vi "ixon get one frame - SubVI.vi"(4 "error in":errorcluster, 5 "Image Height":i32, 6 "Image Width":i32, 7 "Image In":T1) -> (0 "error out":errorcluster, 1 "Image Out":T1)   [LabVIEW 2014]
doc: "Waits till ready and then retireves on frame from an andor camera that has been previously started running a continuous acquisiiton. Uses the GetNewData16 library function."
uses:
  ATMCD32D.DLL
  <vilib>/vision/Image Controls.llb/IMAQ Image.ctl
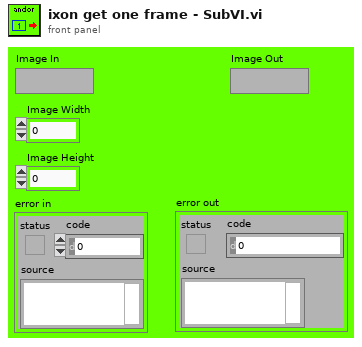
[diagram p1: front panel]
types:
  T1 = typedef "IMAQ Image.ctl" = refnum<image>
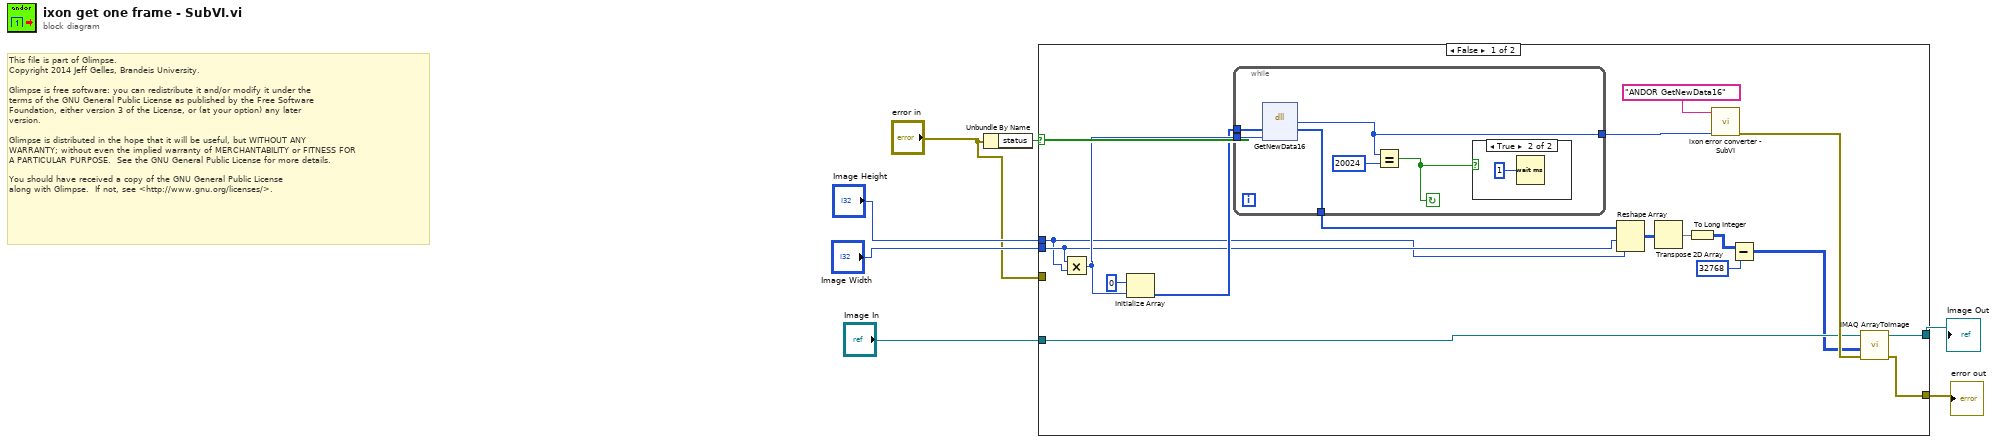
[diagram p0: block diagram]
diagram:
  # "This file is part of Glimpse. \nCopyright 2014 Jeff Gelles, Brandeis University.    \n\nGlimpse is free software: you can redistribute it and/or modify it under the \nterms of the GNU General Public License as published by the Free Software \nFoundation, either version 3 of the License, or (at your option) any later \nversion.\n\nGlimpse is distributed in the hope that it will be useful, but WITHOUT ANY \nWARRANTY; without even the implied warranty of MERCHANTABILITY or FITNESS FOR \nA PARTICULAR PURPOSE.  See the GNU General Public License for more details.\n\nYou should have received a copy of the GNU General Public License\nalong with Glimpse.  If not, see <http://www.gnu.org/licenses/>."
  n1 = Unbundle By Name("error in") -> ("status"=w3:bool)
  n2 = case shown="False" w3 {
    tunnel: "Image Height" -> [w8 _]
    tunnel: "Image Width" -> [w9 _]
    tunnel: "error in" -> [_ w33]
    tunnel: [w17 w33] -> w5
    tunnel: [w15 w32] -> w2
    tunnel: "Image In" -> [w14 w32]
    frame False {
      n3 = Multiply(x=w9, y=w8) -> (x*y=w19:i32)
      n4 = Initialize Array "Initialize Array"(u16 0, w19) -> (w13:u16[])
      n5 = while {
        tunnel: w13 -> [w30]
        tunnel: w19 -> [w29]
        tunnel: [w28] -> w23
        tunnel: [w27] -> w22
        stop <- w25 continue-if-true
        n6 = dll-call lib="ATMCD32D.DLL" fn="GetNewData16" label="Call Library Function\nGetNew data 16"(w30, w29) -> ("return type"=w27:u32, w28:u16[])  [unwired: 4 in, 2 out]
        n7 = Equal?(x=w27, y=u32 20024) -> (x = y?=w25:bool)
        n8 = case shown="True" w25 {
          frame False {
          }
          frame True {
            n9 = Wait (ms)(milliseconds to wait=u32 1) -> ()  [unwired: 1 out]
          }
        }
      }
      n10 = Reshape Array(w23, w9, w8) -> (w21:u16[][])
      n11 = Transpose 2D Array(2D array=w21) -> (transposed array=w18:u16[][])
      n12 = To Long Integer(number=w18) -> (32bit integer=w12:i32[][])
      n13 = call "ixon error converter - SubVI.vi"("Andor error code"=w22, "source"="ANDOR GetNewData16") -> ("error out"=w16:errorcluster)  [unwired: 5 in]
      n14 = Subtract(x=w12, y=32768) -> (x-y=w11:i32[][])
      n15 = call "IMAQ ArrayToImage"("error in (no error)"=w16, "Image Pixels (I16)"=w11, "Image"=w14) -> ("error out"=w17:errorcluster, "Image Out"=w15:T1)  [unwired: 3 in, 4 out]
    }
    frame True {
    }
  }
  "error out" <- w5
  "Image Out" <- w2
